vi "Chirp_Setup.vi"(8 "error in (no error)":errorcluster, 10 "Chirp control":T1={"R external(Ohm)"=150.0, "Chirp Start(Hz)"=0.1, "Chirp Ends(Hz)"=100.0, "Vmin"=0.0, "VInc"=0.2, "Vmax"=0.8, "Chirp T(s)"=0.8}, 11 "ChirpEIS in":refnum<class "ChirpEIS.lvclass">) -> (0 "error out":errorcluster, 3 "ChirpEIS out":refnum<class "ChirpEIS.lvclass">)   [LabVIEW 2014, in "ChirpEIS.lvclass"]
uses:
  ChirpEIS.lvclass
  ChirpEIS.lvclass/ChirpEIS.ctl
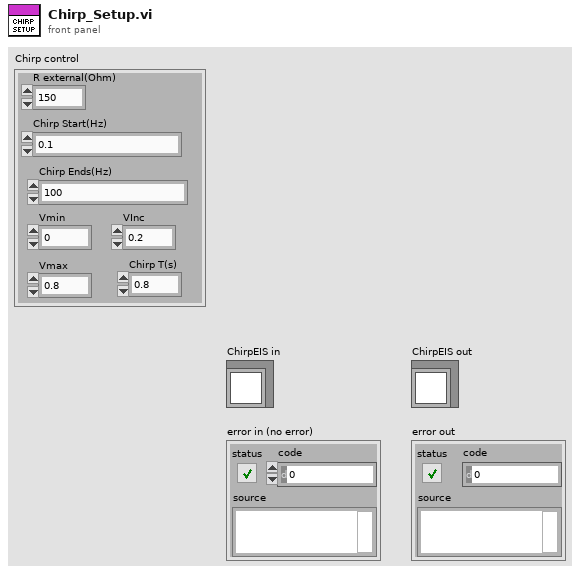
[diagram p1: front panel]
types:
  T1 = cluster{"R external(Ohm)":dbl, "Chirp Start(Hz)":dbl, "Chirp Ends(Hz)":dbl, "Vmin":dbl, "VInc":dbl, "Vmax":dbl, "Chirp T(s)":dbl}
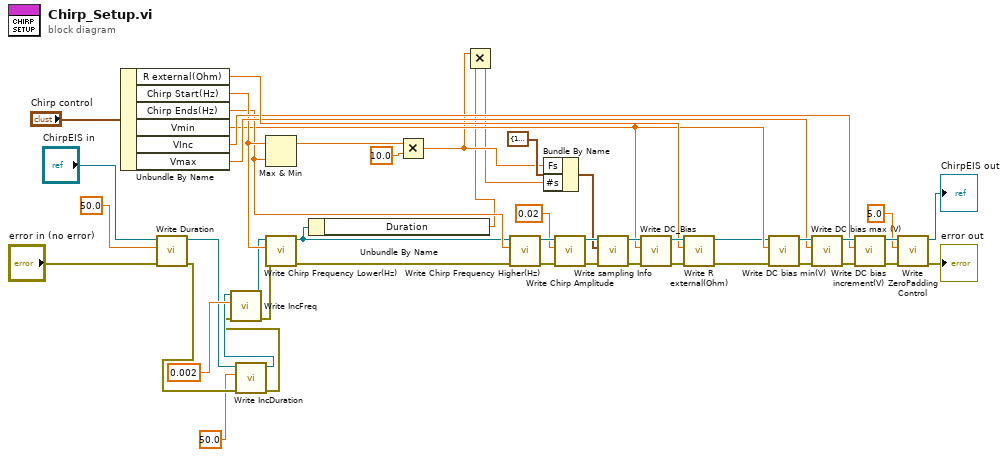
[diagram p0: block diagram]
diagram:
  n1 = Unbundle By Name("Chirp control") -> ("R external(Ohm)"=w37:dbl, "Chirp Start(Hz)"=w30:dbl, "Chirp Ends(Hz)"=w29:dbl, "Vmin"=w18:dbl, "VInc"=w31:dbl, "Vmax"=w32:dbl)
  n2 = call-dynamic "Write Duration.vi"("error in (no error)"="error in (no error)", "Duration"=50.0, "ChirpEIS in"="ChirpEIS in") -> ("error out"=w9:errorcluster, "ChirpEIS out"=w10:refnum<class "ChirpEIS.lvclass">)  [unwired: 7 in]
  n3 = call-dynamic "Write IncDuration.vi"("error in (no error)"=w9, "IncDuration"=50.0, "ChirpEIS in"=w10) -> ("error out"=w7:errorcluster, "ChirpEIS out"=w8:refnum<class "ChirpEIS.lvclass">)  [unwired: 7 in]
  n4 = call-dynamic "Write IncFreq.vi"("error in (no error)"=w7, "IncFreq"=0.002, "ChirpEIS in"=w8) -> ("error out"=w12:errorcluster, "ChirpEIS out"=w13:refnum<class "ChirpEIS.lvclass">)  [unwired: 7 in]
  n5 = Max & Min(x=w30, y=w29) -> (max(x,y)=w27:dbl)  [unwired: 1 out]
  n6 = call-dynamic "Write Chirp Frequency Lower(Hz).vi"("error in (no error)"=w12, "Chirp Frequency Lower(Hz)"=w30, "ChirpEIS in"=w13) -> ("error out"=w44:errorcluster, "ChirpEIS out"=w17:refnum<class "ChirpEIS.lvclass">)  [unwired: 7 in]
  n7 = Unbundle By Name(w17) -> ("Duration"=w4:dbl)
  n8 = Multiply(x=w27, y=10.0) -> (x*y=w5:dbl)
  n9 = Multiply(x=w5, y=w4) -> (x*y=w3:dbl)
  n10 = call-dynamic "Write Chirp Frequency Higher(Hz).vi"("error in (no error)"=w44, "Chirp Frequency Higher(Hz)"=w29, "ChirpEIS in"=w17) -> ("error out"=w45:errorcluster, "ChirpEIS out"=w41:refnum<class "ChirpEIS.lvclass">)  [unwired: 7 in]
  n11 = Bundle By Name(cluster=cluster{"Fs":dbl, "#s":dbl} {"Fs"=100.0, "#s"=10000.0} ("sampling Info"), "Fs"=w5, "#s"=w3) -> (w25:cluster{"Fs":dbl, "#s":dbl})
  n12 = call-dynamic "Write Chirp Amplitude.vi"("error in (no error)"=w45, "Chirp Amplitude"=0.02, "ChirpEIS in"=w41) -> ("error out"=w46:errorcluster, "ChirpEIS out"=w42:refnum<class "ChirpEIS.lvclass">)  [unwired: 7 in]
  n13 = call-dynamic "Write sampling Info.vi"("error in (no error)"=w46, "sampling Info"=w25, "ChirpEIS in"=w42) -> ("error out"=w47:errorcluster, "ChirpEIS out"=w43:refnum<class "ChirpEIS.lvclass">)  [unwired: 7 in]
  n14 = call-dynamic "Write DC_Bias.vi"("error in (no error)"=w47, "DC_Bias"=w18, "ChirpEIS in"=w43) -> ("error out"=w38:errorcluster, "ChirpEIS out"=w39:refnum<class "ChirpEIS.lvclass">)  [unwired: 7 in]
  n15 = call-dynamic "Write R external(Ohm).vi"("error in (no error)"=w38, "R external(Ohm)"=w37, "ChirpEIS in"=w39) -> ("error out"=w1:errorcluster, "ChirpEIS out"=w2:refnum<class "ChirpEIS.lvclass">)  [unwired: 7 in]
  n16 = call-dynamic "Write DC bias min(V) .vi"("error in (no error)"=w1, "DC bias min(V)"=w18, "ChirpEIS in"=w2) -> ("error out"=w34:errorcluster, "ChirpEIS out"=w36:refnum<class "ChirpEIS.lvclass">)  [unwired: 7 in]
  n17 = call-dynamic "Write DC bias max (V).vi"("error in (no error)"=w34, "DC bias max (V)"=w32, "ChirpEIS in"=w36) -> ("error out"=w33:errorcluster, "ChirpEIS out"=w35:refnum<class "ChirpEIS.lvclass">)  [unwired: 7 in]
  n18 = call-dynamic "Write DC bias increment(V).vi"("error in (no error)"=w33, "DC bias increment(V)"=w31, "ChirpEIS in"=w35) -> ("error out"=w23:errorcluster, "ChirpEIS out"=w24:refnum<class "ChirpEIS.lvclass">)  [unwired: 7 in]
  n19 = call-dynamic "Write ZeroPadding Control.vi"("error in (no error)"=w23, "ZeroPadding Control"=5.0, "ChirpEIS in"=w24) -> ("error out"=→"error out":errorcluster, "ChirpEIS out"=→"ChirpEIS out":refnum<class "ChirpEIS.lvclass">)  [unwired: 7 in]
